vi "Tone XCtl Test.vi"() -> ()   [LabVIEW 2015]
uses:
  XControls/Waveform XControls/Tone (G3)/Tone (G3).xctl
  XControls/Waveform XControls/Tone (G3)/Tone.Properties.ctl
  Utility VIs/Controls/KCheckbox/KCheckbox.xctl
panel:
  in  "Array":bool[](array[boolean])
  in  "KCheckbox":bool(xcontrol)
  in  "Apply":bool
  in  "Tone 2":T1={"Frequency (kHz)"=7.0, "Phase (cycles)"=0.0, "Random phase"=FALSE}
  in  "Read":bool
  in  "Tone 1":T1={"Frequency (kHz)"=5.0, "Phase (cycles)"=0.0, "Random phase"=FALSE}
  in  "stop":bool
  in  "Tone (G3)":T2(xcontrol)
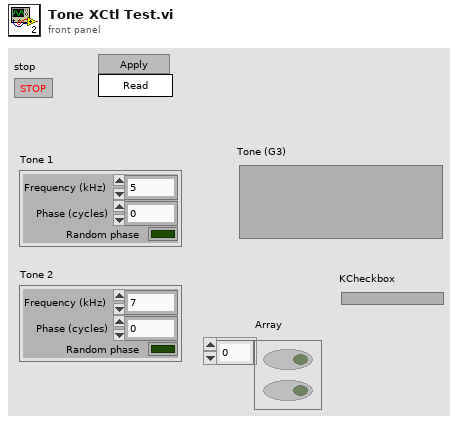
[diagram p1: front panel]
types:
  T1 = typedef "Tone (G3).xctl/Tone.Properties.ctl" = cluster{"Frequency (kHz)":dbl, "Phase (cycles)":dbl, "Random phase":bool}
  T2 = cluster{"Frequency (kHz)":dbl, "Phase (cycles)":dbl, "Random phase":bool}
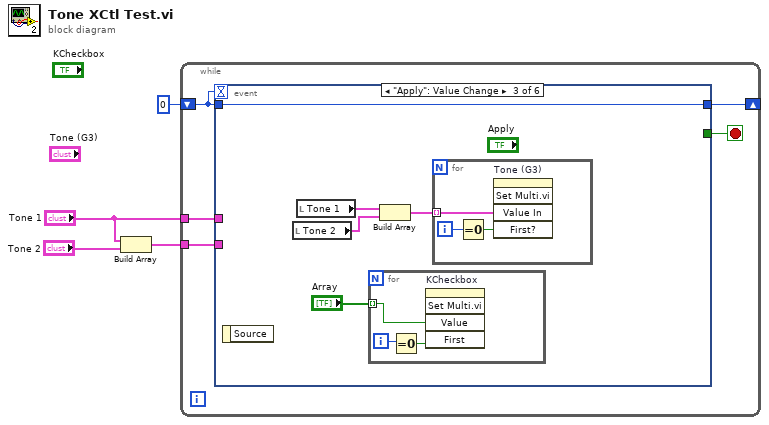
[diagram p0: block diagram]
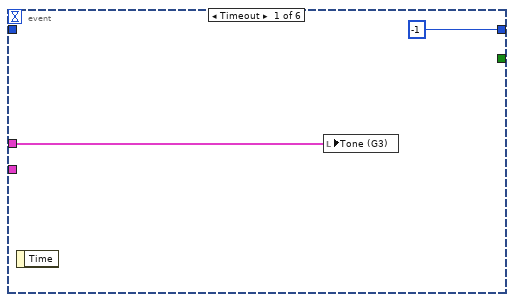
[diagram p2: hidden frame]
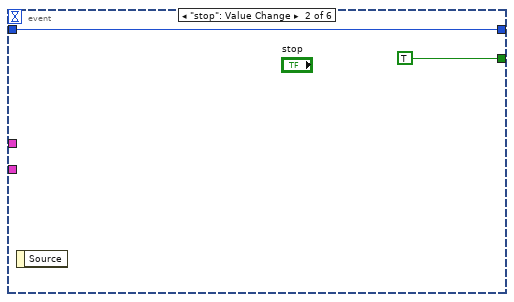
[diagram p3: hidden frame]
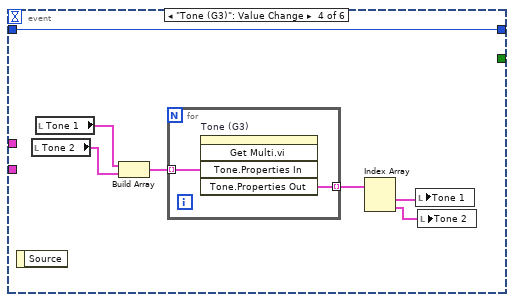
[diagram p4: hidden frame]
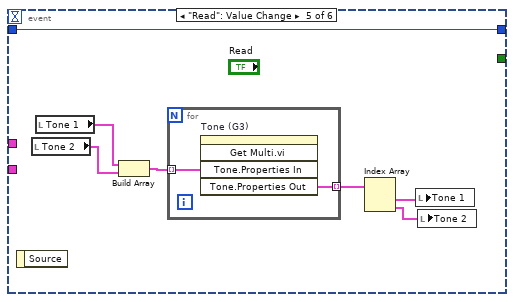
[diagram p5: hidden frame]
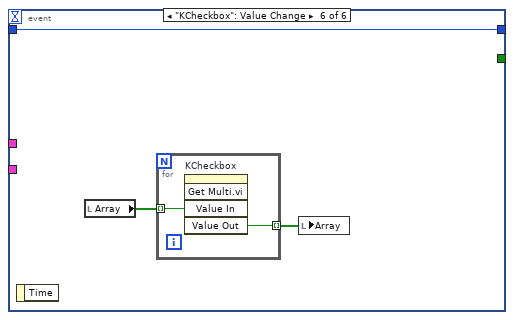
[diagram p6: hidden frame]
diagram:
  n1 = Build Array("Tone 1", "Tone 2") -> (w1:T1[])
  n2 = while {
    shift-right: [w7] -> _
    shift-left: 0 -> [w8]
    tunnel: "Tone 1" -> [w6]
    tunnel: w1 -> [w5]
    stop <- w9 stop-if-true
    n3 = event shown="[2] \"Apply\": Value Change" {
      selector: _ -> [_ _ _ _ _ _]
      dyn-events: _ -> [_ _ _ _ _ _]
      timeout: w8 -> [_ _ _ _ _ _]
      tunnel: [_ TRUE _ _ _ _] -> w9
      tunnel: w8 -> [_ w12 w18 w31 w40 w45]
      tunnel: [-1 w12 w18 w31 w40 w45] -> w7
      tunnel: w6 -> [w10 _ _ _ _ _]
      tunnel: w5 -> [_ _ _ _ _ _]
      event Timeout {
        n4 = event-data() -> ()  [unwired: 1 in, 1 out]
        n5 = local write "Tone (G3)"(w10) -> ()
      }
      event "stop": Value Change {
        n6 = event-data() -> ()  [unwired: 1 in, 1 out]
      }
      event "Apply": Value Change {
        n7 = event-data() -> ()  [unwired: 1 in, 1 out]
        n8 = local read "Tone 2"() -> (w16:T1)
        n9 = local read "Tone 1"() -> (w17:T1)
        n10 = for {
          tunnel: "Array" -> [w19] mode=indexing
          i -> [w21]
          n11 = Equal To 0?(x=w21) -> (x = 0?=w20:bool)
          n12 = invoke on="KCheckbox" class="KCheckbox (strict)" method="Set Multi.vi"("Value"=w19, "First"=w20) -> ()  [unwired: 3 in, 5 out]
        }
        n13 = Build Array(w17, w16) -> (w15:T1[])
        n14 = for {
          tunnel: w15 -> [w24] mode=indexing
          i -> [w22]
          n15 = Equal To 0?(x=w22) -> (x = 0?=w23:bool)
          n16 = invoke on="Tone (G3)" class="Tone (G3) (strict)" method="Set Multi.vi"("Value In"=w24, "First?"=w23) -> ()  [unwired: 3 in, 5 out]
        }
      }
      event "Tone (G3)": Value Change {
        n17 = event-data() -> ()  [unwired: 1 in, 1 out]
        n18 = local read "Tone 2"() -> (w26:T1)
        n19 = local read "Tone 1"() -> (w25:T1)
        n20 = Build Array(w25, w26) -> (w27:T1[])
        n21 = for {
          tunnel: w27 -> [w33] mode=indexing
          tunnel: [w32] -> w30 mode=indexing
          n22 = invoke on="Tone (G3)" class="Tone (G3) (strict)" method="Get Multi.vi"("Tone.Properties In"=w33) -> ("Tone.Properties Out"=w32:T1)  [unwired: 4 in, 4 out]
        }
        n23 = Index Array(array=w30) -> (element #1=w29:T1, element #2=w28:T1)  [unwired: 2 in]
        n24 = local write "Tone 1"(w29) -> ()
        n25 = local write "Tone 2"(w28) -> ()
      }
      event "Read": Value Change {
        n26 = event-data() -> ()  [unwired: 1 in, 1 out]
        n27 = local read "Tone 2"() -> (w35:T1)
        n28 = local read "Tone 1"() -> (w34:T1)
        n29 = Build Array(w34, w35) -> (w36:T1[])
        n30 = for {
          tunnel: w36 -> [w42] mode=indexing
          tunnel: [w41] -> w39 mode=indexing
          n31 = invoke on="Tone (G3)" class="Tone (G3) (strict)" method="Get Multi.vi"("Tone.Properties In"=w42) -> ("Tone.Properties Out"=w41:T1)  [unwired: 4 in, 4 out]
        }
        n32 = Index Array(array=w39) -> (element #1=w38:T1, element #2=w37:T1)  [unwired: 2 in]
        n33 = local write "Tone 1"(w38) -> ()
        n34 = local write "Tone 2"(w37) -> ()
      }
      event "KCheckbox": Value Change {
        n35 = event-data() -> ()  [unwired: 1 in, 1 out]
        n36 = local read "Array"() -> (w44:bool[])
        n37 = for {
          tunnel: w44 -> [w47] mode=indexing
          tunnel: [w46] -> w43 mode=indexing
          n38 = invoke on="KCheckbox" class="KCheckbox (strict)" method="Get Multi.vi"("Value In"=w47) -> ("Value Out"=w46:bool)  [unwired: 4 in, 4 out]
        }
        n39 = local write "Array"(w43) -> ()
      }
    }
  }
